vi "F Dwf Digital In Configure.vi"(8 "error in (no error)":errorcluster, 9 "fStart":i32, 10 "fReconfigure":i32, 11 "hdwf":i32) -> (0 "error out":errorcluster, 3 "function return":i32)   [LabVIEW 2019, in "Olasdwf.lvlib"]
doc: "DWFAPI int FDwfDigitalInConfigure(HDWF hdwf, int fReconfigure, int fStart);"
uses:
  Olasdwf.lvlib
  Windows/System32/dwf.dll
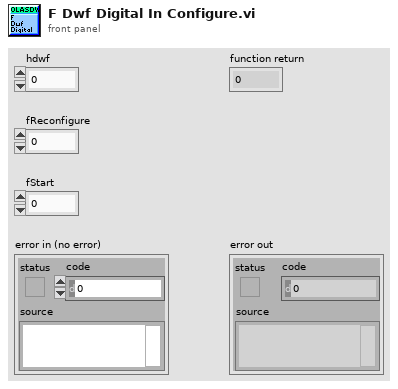
[diagram p1: front panel]
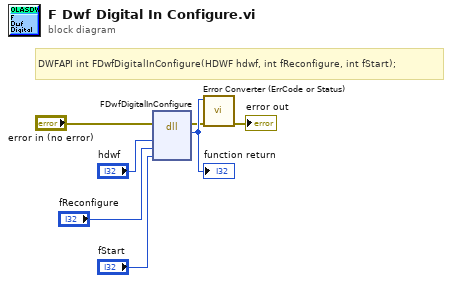
[diagram p0: block diagram]
diagram:
  # "DWFAPI int FDwfDigitalInConfigure(HDWF hdwf, int fReconfigure, int fStart);"
  n1 = dll-call lib="C:/Windows/System32/dwf.*" fn="FDwfDigitalInConfigure"(error in="error in (no error)", "hdwf"="hdwf", "fReconfigure"="fReconfigure", "fStart"="fStart") -> (error out=w2:errorcluster, w7:i32)  [unwired: 5 in, 1 out]
  "function return" <- w7
  n2 = call "Error Converter (ErrCode or Status).vi"("error in (no error)"=w2, "error code"=w7) -> ("error out"=→"error out":errorcluster)  [unwired: 9 in]
